vi "PXI-Find Counter Device.vi"(11 "error in (no error)":errorcluster) -> (4 "Counter Channel":tag, 6 "RefClk.Src":tag="/PXI1Slot4/20MHzTimebase", 8 "Clock Rate":dbl, 10 "Is M-series board":bool, 15 "error out":errorcluster)   [LabVIEW 2020]
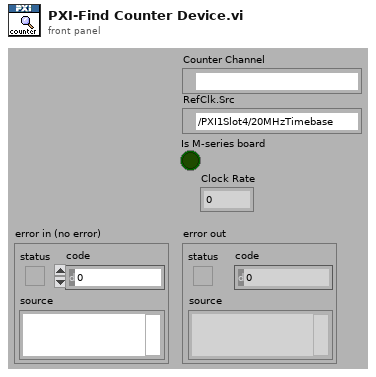
[diagram p1: front panel]
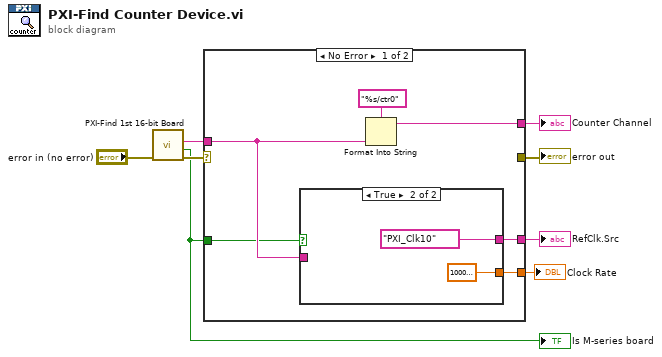
[diagram p0: block diagram]
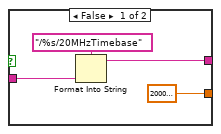
[diagram p2: hidden frame]
diagram:
  n1 = call "PXI-Find 1st 16-bit Board.vi"("error in (no error)"="error in (no error)") -> ("error out"=w3:errorcluster, "Is M-series board"=w2:bool, "DAQmx Device Name"=w5:tag)  [unwired: 8 in]
  "Is M-series board" <- w2
  n2 = case shown="No Error" w3 {
    selector: w3 -> [_ w21]
    tunnel: [w13 _] -> w7
    tunnel: w5 -> [w11 _]
    tunnel: [w12 _] -> w6
    tunnel: [_ w21] -> w4
    tunnel: w2 -> [w10 _]
    tunnel: [w9 _] -> w1
    frame No Error {
      n3 = case shown="True" w10 {
        tunnel: [w16 tag "PXI_Clk10" ("source of ticks")] -> w12
        tunnel: w11 -> [w17 _]
        tunnel: [20000000.0 10000000.0] -> w9
        frame False {
          n4 = Format Into String(format string="/%s/20MHzTimebase", w17) -> (resulting string=w16:string)  [unwired: 2 in, 1 out]
        }
        frame True {
        }
      }
      n5 = Format Into String(format string="%s/ctr0", w11) -> (resulting string=w13:string)  [unwired: 2 in, 1 out]
    }
    frame Error {
    }
  }
  "error out" <- w4
  "Counter Channel" <- w7
  "RefClk.Src" <- w6
  "Clock Rate" <- w1
